vi "Test Matrix Add and Print.vi"() -> ()   [LabVIEW 2014, in "Arduino MatrixMath.lvlib"]
uses:
  <vilib>/Aledyne-TSXperts/Arduino Compatible Compiler for LabVIEW/addons/Arduino MatrixMath/Arduino MatrixMath.lvlib
panel:
  in  "B":sgl[](array[numeric])=[1.0, 2.0, 3.0, 4.0, 5.0, 6.0, 7.0, 8.0]
  out "Error Out":errorcluster
  in  "Error In":errorcluster
  in  "A":sgl[](array[numeric])=[1.0, 2.0, 3.0, 4.0, 5.0, 6.0, 7.0, 8.0]
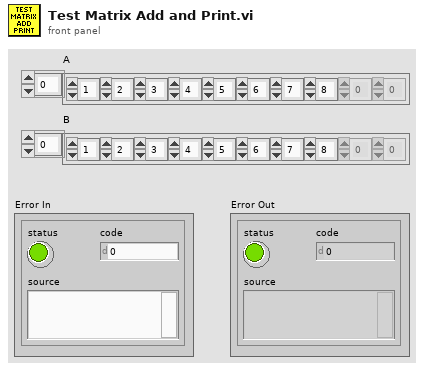
[diagram p1: front panel]
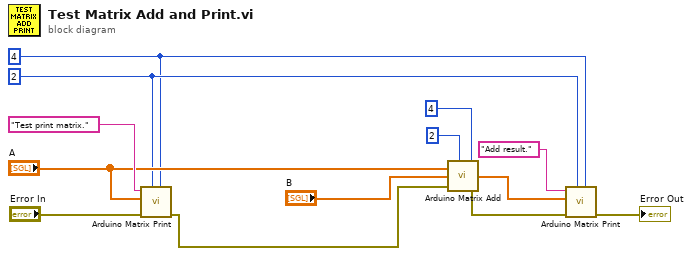
[diagram p0: block diagram]
diagram:
  w1 = u8 4 ("cols num.")
  w2 = u8 2 ("rows num.")
  n1 = call <vilib>:"Arduino Matrix Print.vi"("cols num."=w1, "rows num."=w2, "Error In"="Error In", "A"="A", "Label"="Test print matrix.") -> ("Error Out"=w8:errorcluster)  [unwired: 6 in]
  n2 = call <vilib>:"Arduino Matrix Add.vi"("A"="A", "rows num."=u8 2, "B"="B", "Error In"=w8, "cols num."=u8 4) -> ("A+B"=w4:sgl[], "Error Out"=w6:errorcluster)  [unwired: 1 in]
  n3 = call <vilib>:"Arduino Matrix Print.vi"("cols num."=w1, "rows num."=w2, "Error In"=w6, "A"=w4, "Label"="Add result.") -> ("Error Out"=→"Error Out":errorcluster)  [unwired: 6 in]
